vi "Transform2d_GetXYAngle.vi"(11 "inTRANSFORM":T1={"TRANSLATION"={"X"=0.0, "Y"=0.0}, "ROTATION"={"VALUE"=0.0, "COS"=1.0, "SIN"=0.0}, "xF"=FALSE} {"ROTATION"."SIN" format="%13.4f"; "ROTATION"."COS" format="%13.4f"; "ROTATION"."VALUE" format="%13.4f"; "TRANSLATION"."Y" format="%14.3f"; "TRANSLATION"."X" format="%14.3f"}) -> (1 "Angle":dbl, 2 "Y":dbl format="%14.3f", 3 "X":dbl format="%14.3f")   [LabVIEW 2019, in "Trajectory_Library.lvlib"]
doc: "Returns the X, Y, angle elements of the translation component of the transformation.\n\nParameters:\n - IN TRANSFORM - THis TRANSFORM data structure\n\nReturns:\n - X - The X element of the translational component of the transform.\n - Y - The Y element of the translational component of the transform.\n - angle - The angle element of the translational component of the transform."
uses:
  Trajectory_Library.lvlib
  TypeDef/TRANSFORM2D.ctl
  TypeDef/TRANSLATION2D.ctl
  TypeDef/ROTATION2D.ctl
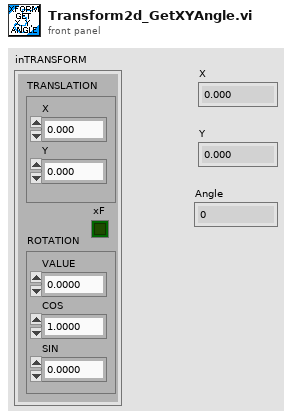
[diagram p1: front panel]
types:
  T1 = typedef "Trajectory_Library.lvlib/TRANSFORM2D.ctl" = cluster{"TRANSLATION":T2, "ROTATION":T3, "xF":bool}
  T2 = typedef "Trajectory_Library.lvlib/TRANSLATION2D.ctl" = cluster{"X":dbl, "Y":dbl}
  T3 = typedef "Trajectory_Library.lvlib/ROTATION2D.ctl" = cluster{"VALUE":dbl, "COS":dbl, "SIN":dbl}
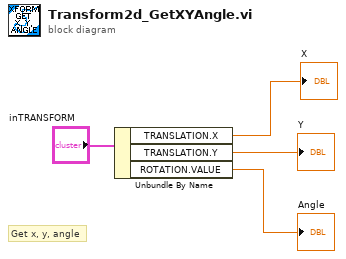
[diagram p0: block diagram]
diagram:
  # "Get x, y, angle"
  n1 = Unbundle By Name("inTRANSFORM") -> ("TRANSLATION.X"=→"X":dbl, "TRANSLATION.Y"=→"Y":dbl, "ROTATION.VALUE"=→"Angle":dbl)
